vi "Mutate_v2_to_v3.vi"(11 "SerializableData_v2":T2) -> (0 "error out":errorcluster, 3 "SerializableData":T1)   [LabVIEW 2019, in "Hulk Hogan.lvclass"]
uses:
  Hulk Hogan.lvclass
  SerializableData_v2.ctl
  SerializableData.ctl
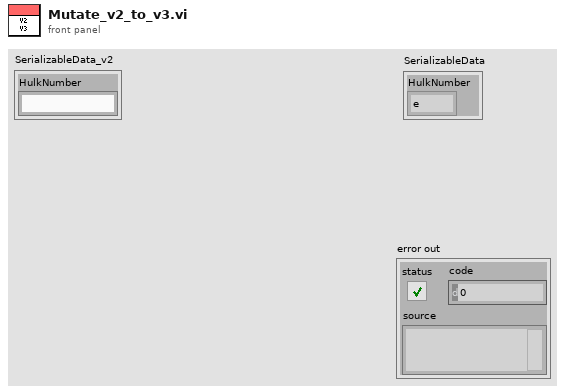
[diagram p1: front panel]
types:
  T1 = typedef "Hulk Hogan.lvclass/SerializableData.ctl" = cluster{"HulkNumber":enum16{"e", "pi", "c"}}
  T2 = typedef "Hulk Hogan.lvclass/SerializableData_v2.ctl" = cluster{"HulkNumber":string}
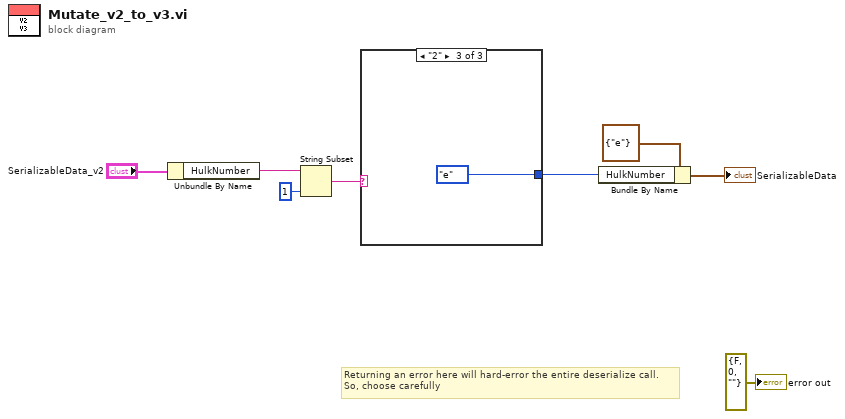
[diagram p0: block diagram]
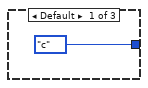
[diagram p2: hidden frame]
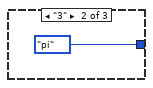
[diagram p3: hidden frame]
diagram:
  # "Returning an error here will hard-error the entire deserialize call.\nSo, choose carefully"
  n1 = Unbundle By Name("SerializableData_v2") -> ("HulkNumber"=w4:string)
  n2 = String Subset(string=w4, length (rest)=1 ("length (rest)")) -> (substring=w2:string)  [unwired: 1 in]
  n3 = case shown="\"2\"" w2 {
    tunnel: [enum16{"e", "pi", "c"}."c" ("HulkNumber") enum16{"e", "pi", "c"}."pi" ("HulkNumber") enum16{"e", "pi", "c"}."e" ("HulkNumber")] -> w1
    frame Default {
    }
    frame "3" {
    }
    frame "2" {
    }
  }
  n4 = Bundle By Name(cluster=T1 {"HulkNumber"=enum."e"} ("SerializableData"), "HulkNumber"=w1) -> (→"SerializableData":T1)
  "error out" <- errorcluster {"status"=FALSE, "code"=0, "source"=""} ("error out")
